vi "Custom Transient Response for Sweep & Single Point.vi"() -> (3 "SourceAdapt Parameters":T1={"Voltage gain bandwidth"=2000.0, "Voltage compensation frequency"=3530.0, "Voltage pole-zero ratio"=2.0, "Current gain bandwidth"=14000.0, "Current compensation frequency"=180000.0, "Current pole-zero ratio"=0.3} {"Current compensation frequency" scale=50.0..1000000.0 scale format="%#_6pHz"; "Voltage compensation frequency" scale=50.0..1000000.0 scale format="%#_6pHz"; "Current pole-zero ratio" scale=0.0625..16.0; "Current gain bandwidth" scale=10.0..1000000.0 scale format="%#_6pHz"; "Voltage pole-zero ratio" scale=0.0625..16.0; "Voltage gain bandwidth" scale=10.0..1000000.0 scale format="%#_6pHz"})   [LabVIEW 2021]
uses:
  controls/SourceAdapt Parameters.ctl
panel:
  in  "SourceAdapt":string="SourceAdapt Parameters"
  in  "Current":string="Current"
  in  "Voltage":string="Voltage"
  in  "Current compensation frequency":dbl(slide)=180000.0 caption="COMP. FREQUENCY" scale=50.0..1000000.0 scale format="%#_6pHz"
  in  "Voltage compensation frequency":dbl(slide)=3530.0 caption="COMP. FREQUENCY" scale=50.0..1000000.0 scale format="%#_6pHz"
  in  "Current pole-zero ratio":dbl(slide)=0.3 caption="POLE-ZERO RATIO" scale=0.0625..16.0
  in  "Current gain bandwidth":dbl(slide)=14000.0 caption="GAIN BANDWIDTH" scale=10.0..1000000.0 scale format="%#_6pHz"
  in  "Voltage pole-zero ratio":dbl(slide)=2.0 caption="POLE-ZERO RATIO" scale=0.0625..16.0
  in  "Voltage gain bandwidth":dbl(slide)=2000.0 caption="GAIN BANDWIDTH" scale=10.0..1000000.0 scale format="%#_6pHz"
  # "Voltage"
  # "Current"
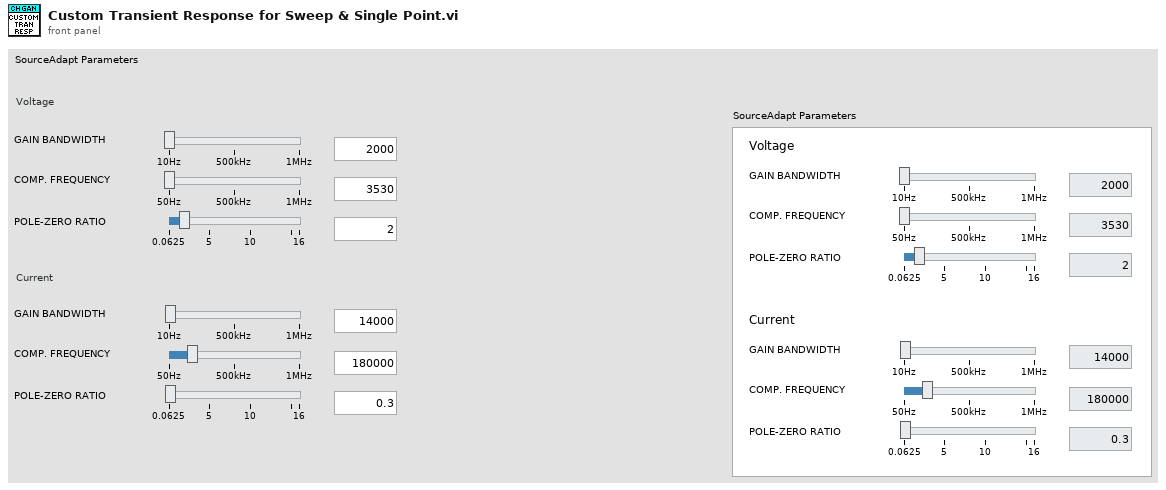
[diagram p1: front panel]
types:
  T1 = typedef "SourceAdapt Parameters.ctl" = cluster{"Voltage gain bandwidth":dbl, "Voltage compensation frequency":dbl, "Voltage pole-zero ratio":dbl, "Current gain bandwidth":dbl, "Current compensation frequency":dbl, "Current pole-zero ratio":dbl}
  T2 = enum32{"Invalid", "Standard", "Closed", "Hidden", "Minimized", "Maximized"}
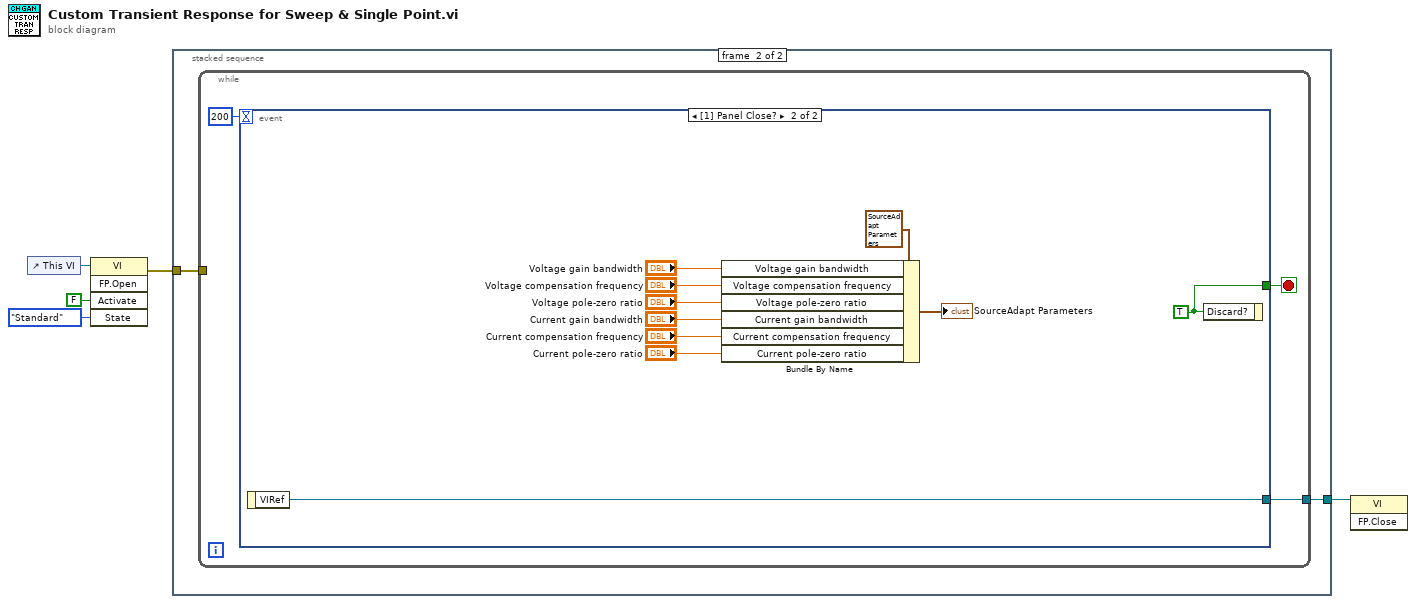
[diagram p0: block diagram]
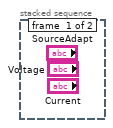
[diagram p2: hidden frame]
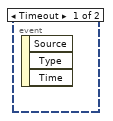
[diagram p3: hidden frame]
diagram:
  n1 = control-ref of="This VI"() -> (w5:refnum<vi>)
  n2 = invoke class="VI" method="FP.Open"(reference=w5, "Activate"=FALSE ("Activate?"), "State"=T2."Standard") -> (error out=w2:errorcluster)  [unwired: 2 in, 4 out]
  n3 = stacked-sequence {
    tunnel: w2 -> [_ w7]
    tunnel: [_ w6] -> w1
    frame #0 {
    }
    frame #1 {
      n4 = while {
        tunnel: [w8] -> w6
        tunnel: w7 -> [_]
        stop <- w10 stop-if-true
        n5 = event shown="[1] Panel Close?" {
          selector: _ -> [_ _]
          dyn-events: _ -> [_ _]
          timeout: 200 -> [_ _]
          tunnel: [_ w19] -> w10
          tunnel: [_ w20] -> w8
          event Timeout {
            n6 = event-data() -> ()  [unwired: 1 in, 3 out]
          }
          event Panel Close? {
            w19 = TRUE ("Discard?")
            n7 = event-data() -> ("VIRef"=w20:refnum<vi>)  [unwired: 1 in]
            n8 = Bundle By Name(cluster=T1 {"Voltage gain bandwidth"=2000.0, "Voltage compensation frequency"=3530.0, "Voltage pole-zero ratio"=2.0, "Current gain bandwidth"=14000.0, "Current compensation frequency"=180000.0, "Current pole-zero ratio"=0.3} ("SourceAdapt Parameters"), "Voltage gain bandwidth"="Voltage gain bandwidth", "Voltage compensation frequency"="Voltage compensation frequency", "Voltage pole-zero ratio"="Voltage pole-zero ratio", "Current gain bandwidth"="Current gain bandwidth", "Current compensation frequency"="Current compensation frequency", "Current pole-zero ratio"="Current pole-zero ratio") -> (→"SourceAdapt Parameters":T1)
            n9 = event-data("Discard?"=w19) -> ()  [unwired: 1 in, 1 out]
          }
        }
      }
    }
  }
  n10 = invoke class="VI" method="FP.Close"(reference=w1) -> ()  [unwired: 2 in, 3 out]
